vi "SubVI_MergeData2.vi"(9 "Data Part 2":dbl[](array[numeric])=[6.06e-39], 10 "Data Part 1":dbl[](array[numeric])=[2.242e-44], 11 "Meas Split Info":T1={"First Signal Index"=0, "Data Type"=2, "Byte Order"=0, "Scaling Offset"=0.0, "Scaling Factor"=1.0, "Numbers of Bytes"=[1, 3]} {"Byte Order" items=["Little Endian", "Big Endian"]; "Data Type" items=["Signed", "Unsigned", "IEEE Float", "Byte Array"]}) -> (3 "Merged Data":dbl[](array[numeric]) format="%#.2f")   [LabVIEW 2019, in "XCP_DaqDtoId.lvlib" / "DAQList.lvclass"]
uses:
  DAQList.lvclass
  TypeDef/MeaSplitInfo2.ctl
panel:
  out "Merged Raw Byte":u8[](array[numeric]) format="%.0x"
  out "Raw Byte Part 2":u8[](array[numeric]) format="%.0x"
  out "Raw Byte Part 1":u8[](array[numeric]) format="%.0x"
  # "The original value is 32.75 but seems like there is some precision lost in the process."
  # "Debug Panel"
  # "0x10"
  # "0xD1 0xFC 0x41"
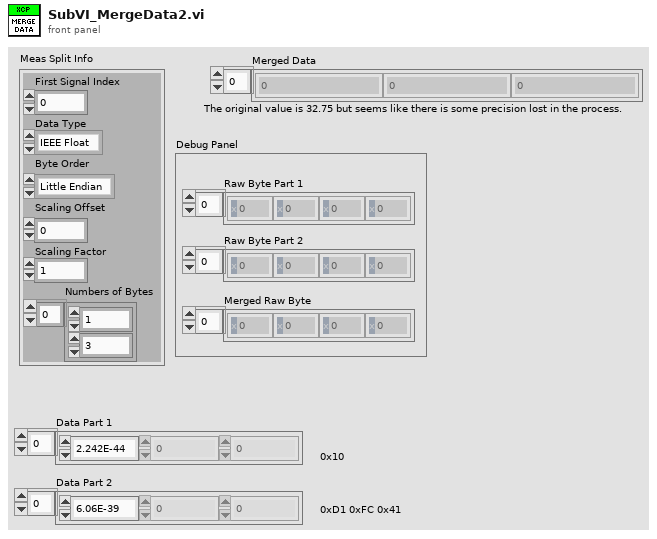
[diagram p1: front panel]
types:
  T1 = typedef "XCP_DaqDtoId.lvlib/DAQList.lvclass/MeaSplitInfo2.ctl" = cluster{"First Signal Index":i32, "Data Type":u32, "Byte Order":u32, "Scaling Offset":dbl, "Scaling Factor":dbl, "Numbers of Bytes":i32[]}
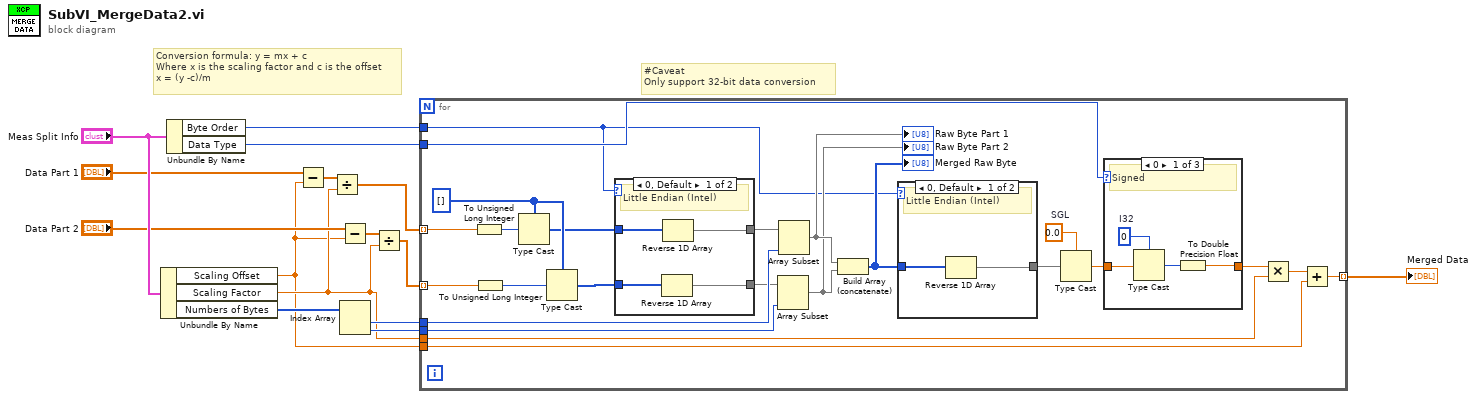
[diagram p0: block diagram]
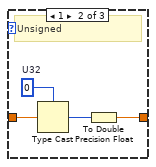
[diagram p4: hidden frame]
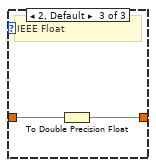
[diagram p5: hidden frame]
diagram:
  # "#Caveat \nOnly support 32-bit data conversion"
  # "Conversion formula: y = mx + c\nWhere x is the scaling factor and c is the offset\nx = (y -c)/m"
  n1 = Unbundle By Name("Meas Split Info") -> ("Scaling Offset"=w3:dbl, "Scaling Factor"=w4:dbl, "Numbers of Bytes"=w10:i32[])
  n2 = Unbundle By Name("Meas Split Info") -> ("Byte Order"=w1:u32, "Data Type"=w2:u32)
  n3 = Subtract(x="Data Part 1", y=w3) -> (x-y=w11:dbl[])
  n4 = Divide(x=w11, y=w4) -> (x/y=w9:dbl[])
  n5 = Subtract(x="Data Part 2", y=w3) -> (x-y=w7:dbl[])
  n6 = Index Array(array=w10) -> (element #1=w8:i32, element #2=w6:i32)  [unwired: 2 in]
  n7 = Divide(x=w7, y=w4) -> (x/y=w5:dbl[])
  n8 = for {
    tunnel: w9 -> [w30] mode=indexing
    tunnel: w8 -> [w39]
    tunnel: w6 -> [w38]
    tunnel: w5 -> [w29] mode=indexing
    tunnel: w4 -> [w34]
    tunnel: w3 -> [w32]
    tunnel: [w31] -> w12 mode=indexing
    tunnel: w2 -> [w21]
    tunnel: w1 -> [w18]
    w28 = u8[] []
    w35 = sgl 0.0  # SGL
    n9 = To Unsigned Long Integer(number=w30) -> (unsigned 32bit integer=w17:u32)
    n10 = To Unsigned Long Integer(number=w29) -> (unsigned 32bit integer=w16:u32)
    n11 = Type Cast(type=w28, x=w17) -> (*(type *) &x=w27:u8[])
    n12 = Type Cast(type=w28, x=w16) -> (*(type *) &x=w24:u8[])
    n13 = case shown="0, Default" w18 {
      tunnel: w27 -> [w43 w45]
      tunnel: [w42 w45] -> w26
      tunnel: [w40 w44] -> w25
      tunnel: w24 -> [w41 w44]
      frame 0, Default {
        # "Little Endian (Intel)"
        n14 = Reverse 1D Array(array=w41) -> (reversed array=w40:u8[])
        n15 = Reverse 1D Array(array=w43) -> (reversed array=w42:u8[])
      }
      frame 1 {
        # "Big Endian (Motorola)"
      }
    }
    n16 = Array Subset(array=w25, length=w38) -> (w36:u8[])  [unwired: 1 in]
    "Raw Byte Part 2" <- w36
    n17 = Array Subset(array=w26, length=w39) -> (w37:u8[])  [unwired: 1 in]
    "Raw Byte Part 1" <- w37
    n18 = Build Array (concatenate)(w37, w36) -> (w20:u8[])
    "Merged Raw Byte" <- w20
    n19 = case shown="0, Default" w18 {
      tunnel: w20 -> [w47 w48]
      tunnel: [w46 w48] -> w19
      frame 0, Default {
        # "Little Endian (Intel)"
        n20 = Reverse 1D Array(array=w47) -> (reversed array=w46:u8[])
      }
      frame 1 {
        # "Big Endian (Motorola)"
      }
    }
    n21 = Type Cast(type=w35, x=w19) -> (*(type *) &x=w23:sgl)
    n22 = case shown="0" w21 {
      tunnel: w23 -> [w51 w54 w58]
      tunnel: [w49 w53 w57] -> w22
      frame 0 {
        w50 = 0  # I32
        # "Signed"
        n23 = Type Cast(type=w50, x=w51) -> (*(type *) &x=w52:i32)
        n24 = To Double Precision Float(number=w52) -> (double precision float=w49:dbl)
      }
      frame 1 {
        w55 = u32 0  # U32
        # "Unsigned"
        n25 = Type Cast(type=w55, x=w54) -> (*(type *) &x=w56:u32)
        n26 = To Double Precision Float(number=w56) -> (double precision float=w53:dbl)
      }
      frame 2, Default {
        # "IEEE Float"
        n27 = To Double Precision Float(number=w58) -> (double precision float=w57:dbl)
      }
    }
    n28 = Multiply(x=w22, y=w34) -> (x*y=w33:dbl)
    n29 = Add(x=w33, y=w32) -> (x+y=w31:dbl)
  }
  "Merged Data" <- w12
